vi "Fuente de poder_Init.vi"(0 "object in":refnum<class "Fuente de poder.lvclass">, 5 "error in (no error)":errorcluster) -> (14 "object out":refnum<class "Fuente de poder.lvclass">, 19 "error out":errorcluster)   [LabVIEW 2020, in "Fuente de poder.lvclass"]
uses:
  Fuente de poder.lvclass
  Fuente de poder.lvclass/Fuente de poder.ctl
  Contador Actor_class/Contador Actor.lvclass
  D:/Storage/Source Code/Clase AF/ClaseAF/11 OOP Interfaces/Instrumento/Instrumento.lvclass
  D:/Storage/Source Code/Clase AF/ClaseAF/11 OOP Interfaces/Fuente de poder_class/Fuente de poder.lvclass
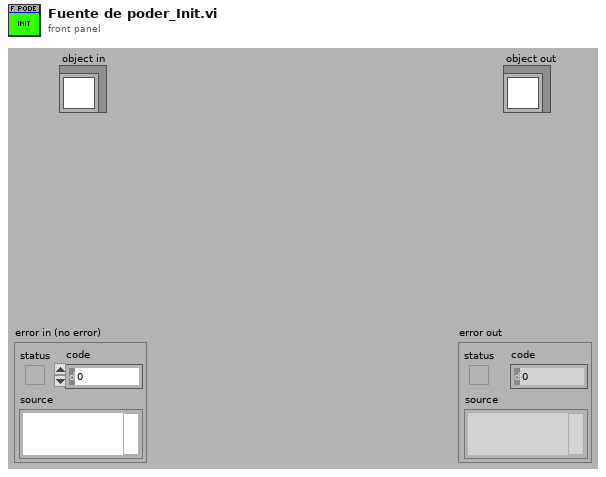
[diagram p1: front panel]
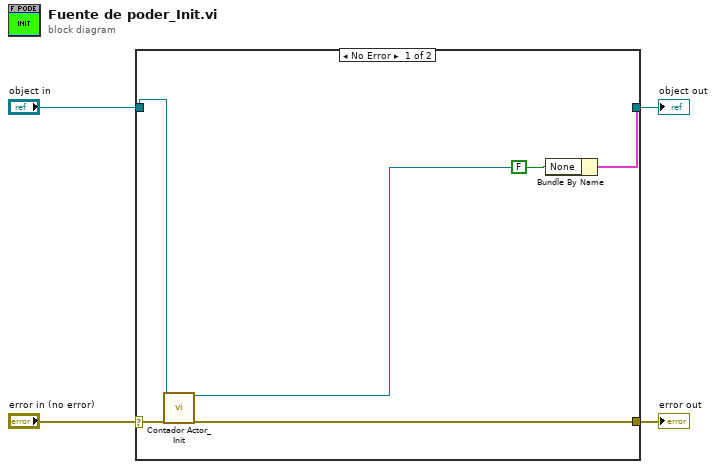
[diagram p0: block diagram]
diagram:
  n1 = case shown="No Error" "error in (no error)" {
    selector: "error in (no error)" -> [w8 w11]
    tunnel: [w10 w12] -> w4
    tunnel: "object in" -> [w6 w12]
    tunnel: [w7 w11] -> w1
    frame No Error {
      n2 = call "Contador Actor_Init.vi"("object in"=w6, "error in (no error)"=w8) -> ("object out"=w5:refnum<class "Contador Actor.lvclass">, "error out"=w7:errorcluster)  [unwired: 16 in]
      n3 = Bundle By Name(cluster=w5, "None"=FALSE) -> (w10:cluster{})
    }
    frame Error {
    }
  }
  "object out" <- w4
  "error out" <- w1
